vi "20TMonitor.vi"() -> ()   [LabVIEW 2019]
uses:
  Utility/Monitor Communication/Gustav/20T_Cluster.ctl
  Instrument_Setup.vi
  Global/Global Variables/Data_Display_global.vi
  Equipment/Mercury iXX/Public/Libraries/Magnet/Open/Open Magnet Device.vi
  Equipment/Mercury iXX/Public/Libraries/Magnet/Signals/Read/Persistant Field (Read).vi
  Equipment/Mercury iXX/Public/Libraries/Magnet/Signals/Read/Field (Read).vi
  Equipment/Mercury iXX/Public/Libraries/Magnet/Signals/Read/Voltage (Read).vi
  Equipment/Mercury iXX/Public/Libraries/Lambda/Open/Open Lambda Device.vi
  Equipment/Mercury iXX/Public/Libraries/Lambda/Signals/Read/Lambda Pressure (Read).vi
  Equipment/Mercury iXX/Public/Libraries/Lambda/Signals/Read/Lambda Valve Open Percent (Read).vi
  Equipment/Mercury iXX/Public/Libraries/Magnet/Signals/Read/Switch Heater Status (Read).vi
  Equipment/Mercury iXX/Public/Libraries/Magnet/Configuration/Read/PSU Action Status (Read).vi
  Equipment/Mercury iXX/Public/Libraries/Magnet/Configuration/Read/PSU Status (Read).vi
  Equipment/Mercury iXX/Public/Libraries/Magnet/Signals/Read/Target Field (Read).vi
  Equipment/Mercury iXX/Public/Libraries/Magnet/Signals/Read/Target Field Rate (Read).vi
  Equipment/Mercury iXX/Public/Libraries/Temperature/Open/Open Temperature Device.vi
  Equipment/Mercury iXX/Public/Libraries/Temperature/Signals/Read/Temperature (Read).vi
  Utility/Monitor Communication/sub-vis/20T_Open_Queue.vi
  Utility/Gustav/20T_Set_Rate.vi
  Utility/Gustav/20T_Go_To_Set.vi
  Utility/Gustav/20T_Go_To_Zero.vi
  Utility/Gustav/20T_Set_Hold.vi
  Utility/Gustav/20T_Set_Clamp.vi
  Equipment/Mercury iXX/Mercury iXX.lvlib
  Equipment/Mercury iXX/Public/Libraries/Magnet.lvlib
  Equipment/Mercury iXX/Public/Libraries/Lambda.lvlib
  Equipment/Mercury iXX/Public/Libraries/Temperature.lvlib
panel:
  out "20 T Magnet control":T1={"Clamp"=FALSE, "Switch Heater"=FALSE, "Go to Zero"=FALSE, "Go to set"=FALSE, "Go to Hold"=FALSE, "Clamped"=FALSE, "Hold"=FALSE, "Set"=FALSE, "Zero"=FALSE, "Magnet (T)"=0.0, "Leads (T)"=0.0, "Magnet T (K)"=3.4572, "Switch"=FALSE, "Target Field (T)"=3.4572, "Field Setpoint (T)"=3.4572, "Rate Setpoint (T/min)"=0.0, "Set Rate"=FALSE, "Rate\n(T/min) "=3.4572, "lambda NV (%)"=3.4572, "lambda p (mbar)"=3.4572, "lambda-Control"=FALSE, "Activate lambda control"=FALSE, "lambda NV  SP"=3.4572, "Set lambda NV"=FALSE, "PSU Status"="", "PSU\nVoltage"=3.4572} {"PSU\nVoltage" format="%.3f"; "lambda NV  SP" format="%.1f"; "lambda p (mbar)" format="%.1f"; "lambda NV (%)" scale=0.0..100.0; "Rate\n(T/min)" format="%.3f"; "Rate Setpoint (T/min)" format="%6.3f"; "Field Setpoint (T)" format="%6.3f"; "Target Field (T)" format="%.3f"; "Magnet T (K)" format="%4.3f"; "Leads (T)" format="%.3f"; "Magnet (T)" format="%.3g"}
  # "20 T"
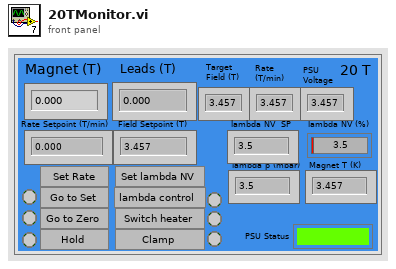
[diagram p1: front panel]
types:
  T1 = typedef "20T_Cluster.ctl" = cluster{"Clamp":bool, "Switch Heater":bool, "Go to Zero":bool, "Go to set":bool, "Go to Hold":bool, "Clamped":bool, "Hold":bool, "Set":bool, "Zero":bool, "Magnet (T)":dbl, "Leads (T)":dbl, "Magnet T (K)":dbl, "Switch":bool, "Target Field (T)":dbl, "Field Setpoint (T)":dbl, "Rate Setpoint (T/min)":dbl, "Set Rate":bool, "Rate\n(T/min) ":dbl, "lambda NV (%)":dbl, "lambda p (mbar)":dbl, "lambda-Control":bool, "Activate lambda control":bool, "lambda NV  SP":dbl, "Set lambda NV":bool, "PSU Status":string, "PSU\nVoltage":dbl}
  T2 = typedef "Mercury iXX.lvlib/Mercury Reference.ctl" = cluster{"Comms":refnum<visa-resource-name>, "Device ID":string[], "Comms Layer":T3, "Command":string, "Query reference":T4}
  T3 = typedef "Mercury iXX.lvlib/Comms Transport Layer.ctl" = enum16{"Ethernet TCP/IP", "USB", "ISOBus - RS-232", "GPIB"}
  T4 = typedef "Mercury iXX.lvlib/Query Dynamic Reference.ctl" = refnum<vi>
  T5 = typedef "Mercury iXX.lvlib/Magnet.lvlib/PSU Actions.ctl" = string
  T6 = typedef "20T_Control.ctl" = cluster{"Clamp":bool, "Switch Heater":bool, "Go to Zero":bool, "Go to Set":bool, "Go to Hold":bool, "Field Setpoint (T)":dbl, "Rate Setpoint (T/min)":dbl, "Set Rate":bool, "Activate lambda control":bool, "Set lambda NV":bool, "lambda NV  SP":dbl}
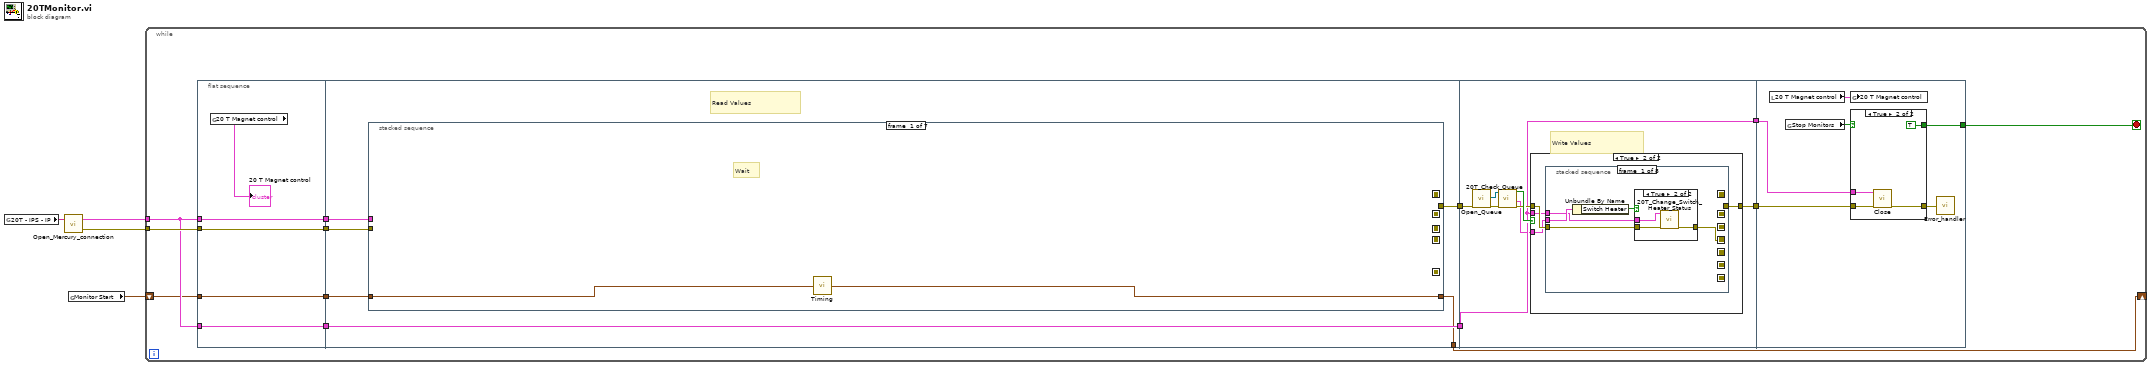
[diagram p0: block diagram]
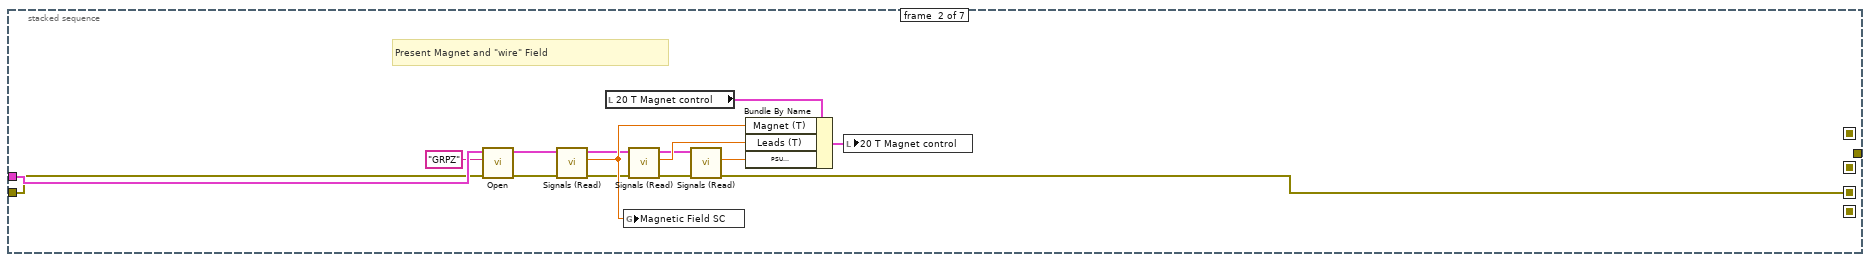
[diagram p2: hidden frame]
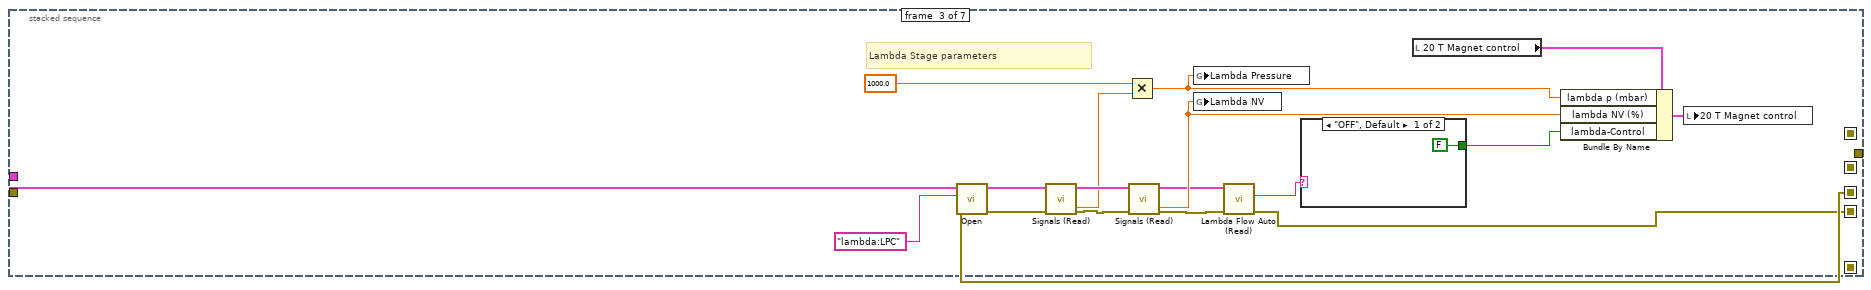
[diagram p3: hidden frame]
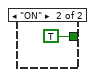
[diagram p4: hidden frame]
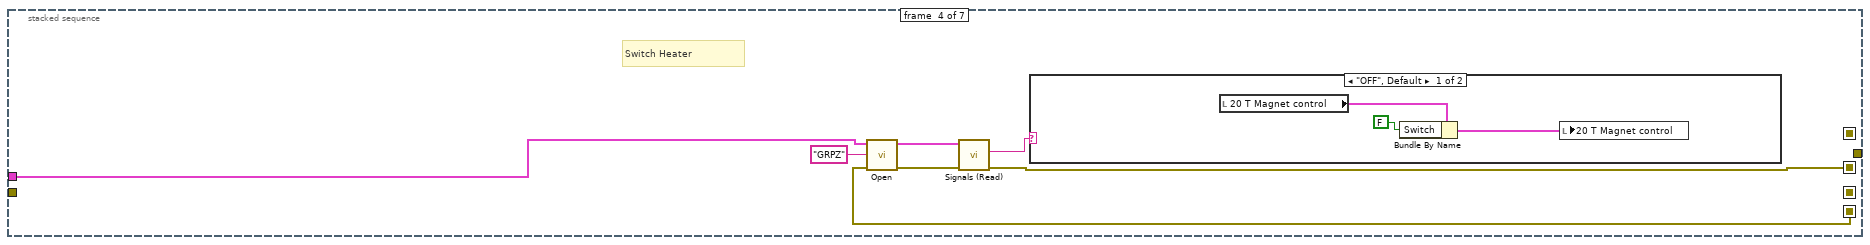
[diagram p5: hidden frame]
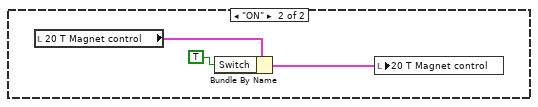
[diagram p6: hidden frame]
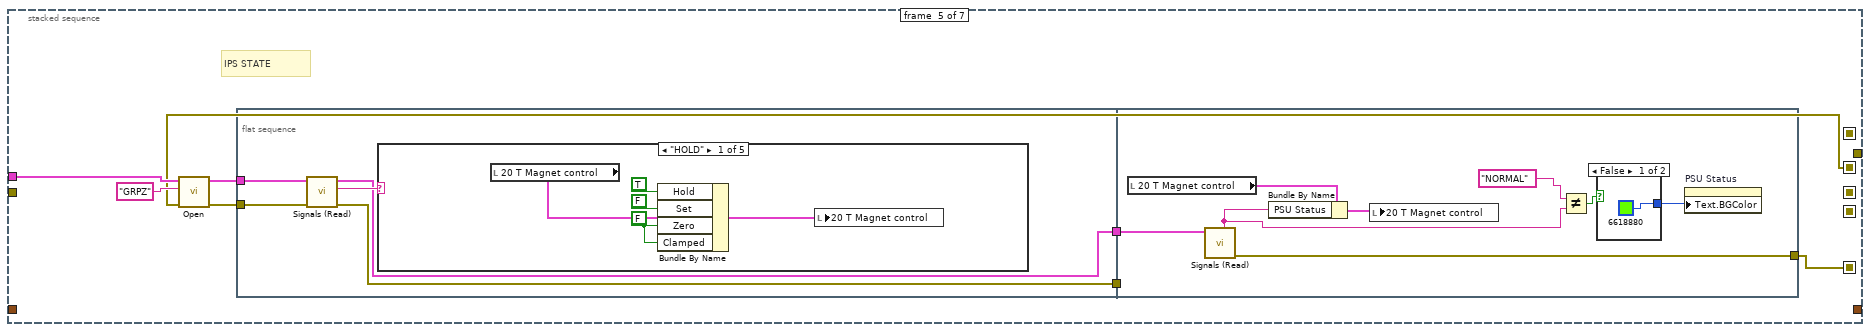
[diagram p7: hidden frame]
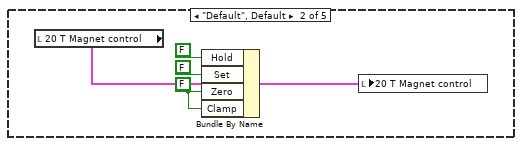
[diagram p8: hidden frame]
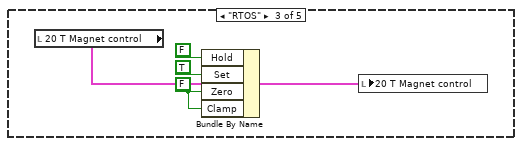
[diagram p9: hidden frame]
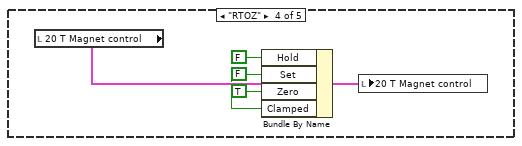
[diagram p10: hidden frame]
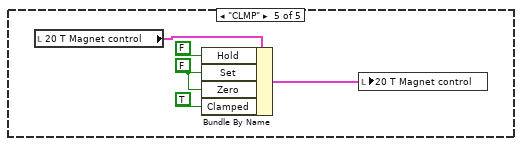
[diagram p11: hidden frame]
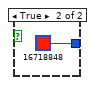
[diagram p12: hidden frame]
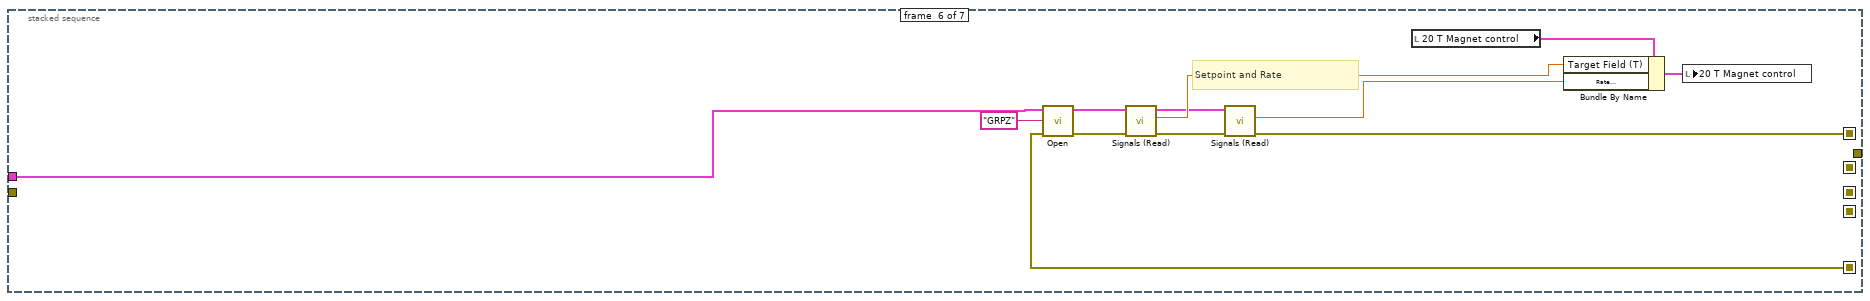
[diagram p13: hidden frame]
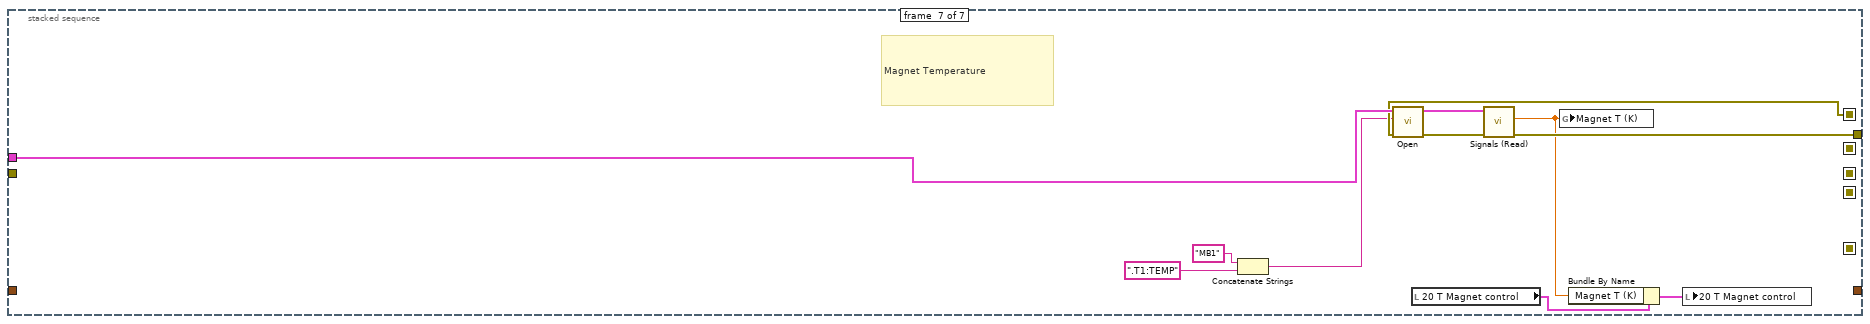
[diagram p14: hidden frame]
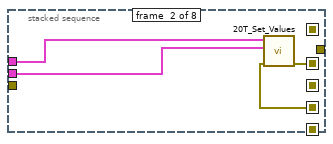
[diagram p17: hidden frame]
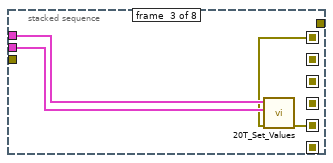
[diagram p18: hidden frame]
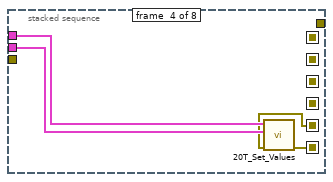
[diagram p19: hidden frame]
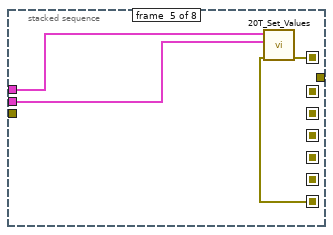
[diagram p20: hidden frame]
diagram:
  n1 = global read "Instrument_Setup.vi" "20T - IPS - IP"() -> (w4:string)
  n2 = call "Open_Mercury_connection.vi"("IP Address"=w4) -> ("error out"=w3:errorcluster, "Mercury Reference Out"=w2:T2)  [unwired: 1 in]
  n3 = global read "Data_Display_global.vi" "Monitor Start"() -> (w1:timestamp)
  n4 = while {
    tunnel: w3 -> [w15]
    tunnel: w2 -> [w14]
    shift-right: [w11] -> _
    shift-left: w1 -> [w12]
    stop <- w17 stop-if-true
    n5 = flat-sequence {
      tunnel: w12 -> [w19]
      tunnel: w14 -> [w20]
      tunnel: w14 -> [w21]
      tunnel: w15 -> [w22]
      tunnel: [w22] -> w10
      tunnel: [w21] -> w9
      tunnel: [w20] -> w8
      tunnel: [w19] -> w7
      tunnel: [w28] -> w16
      tunnel: [w25] -> w13
      tunnel: [w24] -> w11
      tunnel: w10 -> [w27]
      tunnel: w9 -> [w26]
      tunnel: w8 -> [w25]
      tunnel: w7 -> [w23]
      tunnel: [w151] -> w6
      tunnel: [w157] -> w5
      tunnel: w16 -> [w154]
      tunnel: w13 -> [w151]
      tunnel: w6 -> [w204]
      tunnel: w5 -> [w203]
      tunnel: [w201] -> w17
      frame #0 {
        n6 = global read "Data_Display_global.vi" "20 T Magnet control"() -> (→"20 T Magnet control":T1)
      }
      frame #1 {
        # "Read Values"
        n7 = stacked-sequence {
          seq-local: [_ w34 _ _ _ _ _] -> [_ _ w61 _ _ _ _]
          seq-local: [_ _ w47 _ _ _ _] -> [_ _ _ w68 _ _ _]
          seq-local: [_ _ _ w67 _ _ _] -> [_ _ _ _ w82 _ _]
          seq-local: [_ _ _ _ w79 _ _] -> [_ _ _ _ _ w134 _]
          seq-local: [_ _ _ _ _ w129 _] -> [_ _ _ _ _ _ w143]
          tunnel: w26 -> [_ w43 w51 w70 w84 w136 w147]
          tunnel: w27 -> [_ w42 _ _ _ _ _]
          tunnel: [_ _ _ _ _ _ w146] -> w28
          tunnel: [w30 _ _ _ _ _ _] -> w24
          tunnel: w23 -> [w29 _ _ _ _ _ _]
          frame #0 {
            # "Wait"
            n8 = call "Timing.vi"("start time (s)"=w29) -> ("last reading (s)"=w30:timestamp)
          }
          frame #1 {
            # "Present Magnet and \"wire\" Field"
            n9 = call-poly "Open.vi"("error in (no error)"=w42, "Device Identifier"="GRPZ", "Mercury Reference In"=w43) -> ("error out"=w45:errorcluster, "Mercury Reference Out"=w44:T2)  [unwired: 1 in, 6 out]
            n10 = call-poly "Signals (Read).vi"("error in"=w45, "Mercury Reference In"=w44) -> ("error out"=w35:errorcluster, "Persistant Field"=w38:dbl, "Mercury Reference Out"=w37:T2)  [unwired: 5 in, 2 out]
            n11 = local read "20 T Magnet control"() -> (w40:T1)
            n12 = global write "Data_Display_global.vi" "Magnetic Field SC"(w38) -> ()
            n13 = call-poly "Signals (Read).vi"("error in"=w35, "Mercury Reference In"=w37) -> ("error out"=w33:errorcluster, "Field"=w36:dbl, "Mercury Reference Out"=w32:T2)  [unwired: 5 in, 2 out]
            n14 = call-poly "Signals (Read).vi"("error in"=w33, "Mercury Reference In"=w32) -> ("error out"=w34:errorcluster, "Voltage"=w31:dbl)  [unwired: 5 in, 3 out]
            n15 = Bundle By Name(cluster=w40, "Magnet (T)"=w38, "Leads (T)"=w36, "PSU\nVoltage"=w31) -> (w39:T1)
            n16 = local write "20 T Magnet control"(w39) -> ()
          }
          frame #2 {
            # "Lambda Stage parameters"
            n17 = call-poly "Open.vi"("error in (no error)"=w61, "Device Identifier"="lambda:LPC", "Mercury Reference In"=w51) -> ("error out"=w63:errorcluster, "Mercury Reference Out"=w62:T2)  [unwired: 1 in, 6 out]
            n18 = call-poly "Signals (Read).vi"("error in"=w63, "Mercury Reference In"=w62) -> ("error out"=w58:errorcluster, "Pressure"=w55:dbl, "Mercury Reference Out"=w57:T2)  [unwired: 5 in, 2 out]
            n19 = Multiply(x=1000.0, y=w55) -> (x*y=w52:dbl)
            n20 = call-poly "Signals (Read).vi"("error in"=w58, "Mercury Reference In"=w57) -> ("error out"=w48:errorcluster, "Open"=w53:dbl, "Mercury Reference Out"=w49:T2)  [unwired: 5 in, 2 out]
            n21 = global write "Data_Display_global.vi" "Lambda Pressure"(w52) -> ()
            n22 = global write "Data_Display_global.vi" "Lambda NV"(w53) -> ()
            n23 = call "Lambda Flow Auto (Read).vi"("error in"=w48, "Mercury Reference In"=w49) -> ("error out"=w47:errorcluster, "Lambda Auto"=w46:string)  [unwired: 6 in, 2 out]
            n24 = case shown="\"OFF\", Default" w46 {
              tunnel: [FALSE TRUE] -> w50
              frame "OFF", Default {
              }
              frame "ON" {
              }
            }
            n25 = local read "20 T Magnet control"() -> (w60:T1)
            n26 = Bundle By Name(cluster=w60, "lambda p (mbar)"=w52, "lambda NV (%)"=w53, "lambda-Control"=w50) -> (w59:T1)
            n27 = local write "20 T Magnet control"(w59) -> ()
          }
          frame #3 {
            # "Switch Heater"
            n28 = call-poly "Open.vi"("error in (no error)"=w68, "Device Identifier"="GRPZ", "Mercury Reference In"=w70) -> ("error out"=w72:errorcluster, "Mercury Reference Out"=w71:T2)  [unwired: 1 in, 6 out]
            n29 = call-poly "Signals (Read).vi"("error in"=w72, "Mercury Reference In"=w71) -> ("error out"=w67:errorcluster, "Switch Heater Status"=w66:string)  [unwired: 6 in, 2 out]
            n30 = case shown="\"OFF\", Default" w66 {
              frame "OFF", Default {
                n31 = local read "20 T Magnet control"() -> (w73:T1)
                n32 = Bundle By Name(cluster=w73, "Switch"=FALSE) -> (w75:T1)
                n33 = local write "20 T Magnet control"(w75) -> ()
              }
              frame "ON" {
                n34 = local read "20 T Magnet control"() -> (w77:T1)
                n35 = Bundle By Name(cluster=w77, "Switch"=TRUE) -> (w78:T1)
                n36 = local write "20 T Magnet control"(w78) -> ()
              }
            }
          }
          frame #4 {
            # "IPS STATE"
            n37 = call-poly "Open.vi"("error in (no error)"=w82, "Device Identifier"="GRPZ", "Mercury Reference In"=w84) -> ("error out"=w86:errorcluster, "Mercury Reference Out"=w85:T2)  [unwired: 1 in, 6 out]
            n38 = flat-sequence {
              tunnel: w86 -> [w91]
              tunnel: w85 -> [w90]
              tunnel: [w88] -> w81
              tunnel: [w87] -> w80
              tunnel: w81 -> [w123]
              tunnel: w80 -> [_]
              tunnel: [w124] -> w79
              frame #0 {
                n39 = call-poly "Signals (Read).vi"("error in"=w91, "Mercury Reference In"=w90) -> ("error out"=w87:errorcluster, "PSU Act Stat"=w89:T5, "Mercury Reference Out"=w88:T2)  [unwired: 6 in, 1 out]
                n40 = case shown="\"HOLD\"" w89 {
                  frame "HOLD" {
                    w92 = FALSE
                    n41 = local read "20 T Magnet control"() -> (w96:T1)
                    n42 = Bundle By Name(cluster=w96, "Hold"=TRUE, "Set"=FALSE, "Zero"=w92, "Clamped"=w92) -> (w95:T1)
                    n43 = local write "20 T Magnet control"(w95) -> ()
                  }
                  frame "Default", Default {
                    w97 = FALSE
                    n44 = local read "20 T Magnet control"() -> (w101:T1)
                    n45 = Bundle By Name(cluster=w101, "Hold"=FALSE, "Set"=FALSE, "Zero"=w97, "Clamp"=w97) -> (w100:T1)
                    n46 = local write "20 T Magnet control"(w100) -> ()
                  }
                  frame "RTOS" {
                    w102 = FALSE
                    n47 = local read "20 T Magnet control"() -> (w106:T1)
                    n48 = Bundle By Name(cluster=w106, "Hold"=FALSE, "Set"=TRUE, "Zero"=w102, "Clamp"=w102) -> (w105:T1)
                    n49 = local write "20 T Magnet control"(w105) -> ()
                  }
                  frame "RTOZ" {
                    w107 = FALSE
                    n50 = local read "20 T Magnet control"() -> (w111:T1)
                    n51 = Bundle By Name(cluster=w111, "Hold"=FALSE, "Set"=w107, "Zero"=TRUE, "Clamped"=w107) -> (w110:T1)
                    n52 = local write "20 T Magnet control"(w110) -> ()
                  }
                  frame "CLMP" {
                    w112 = FALSE
                    n53 = local read "20 T Magnet control"() -> (w116:T1)
                    n54 = Bundle By Name(cluster=w116, "Hold"=FALSE, "Set"=w112, "Zero"=w112, "Clamped"=TRUE) -> (w115:T1)
                    n55 = local write "20 T Magnet control"(w115) -> ()
                  }
                }
              }
              frame #1 {
                n56 = local read "20 T Magnet control"() -> (w122:T1)
                n57 = call-poly "Signals (Read).vi"("Mercury Reference In"=w123) -> ("error out"=w124:errorcluster, "Status"=w120:string)  [unwired: 5 in, 4 out]
                n58 = Bundle By Name(cluster=w122, "PSU Status"=w120) -> (w121:T1)
                n59 = local write "20 T Magnet control"(w121) -> ()
                n60 = Not Equal?(x="NORMAL", y=w120) -> (x != y?=w118:bool)
                n61 = case shown="False" w118 {
                  tunnel: [u32 6618880 u32 16718848] -> w117
                  frame False {
                  }
                  frame True {
                  }
                }
                n62 = property on="PSU Status" class="Str"("Text.BGColor"=w117) -> ()  [unwired: 2 in, 2 out]
              }
            }
          }
          frame #5 {
            # "Setpoint and Rate"
            n63 = call-poly "Open.vi"("error in (no error)"=w134, "Device Identifier"="GRPZ", "Mercury Reference In"=w136) -> ("error out"=w138:errorcluster, "Mercury Reference Out"=w137:T2)  [unwired: 1 in, 6 out]
            n64 = call-poly "Signals (Read).vi"("error in"=w138, "Mercury Reference In"=w137) -> ("error out"=w130:errorcluster, "Target Field"=w131:dbl, "Mercury Reference Out"=w128:T2)  [unwired: 5 in, 2 out]
            n65 = call-poly "Signals (Read).vi"("error in"=w130, "Mercury Reference In"=w128) -> ("error out"=w129:errorcluster, "Target Field Rate"=w127:dbl)  [unwired: 5 in, 3 out]
            n66 = local read "20 T Magnet control"() -> (w133:T1)
            n67 = Bundle By Name(cluster=w133, "Target Field (T)"=w131, "Rate\n(T/min)"=w127) -> (w132:T1)
            n68 = local write "20 T Magnet control"(w132) -> ()
          }
          frame #6 {
            # "Magnet Temperature"
            n69 = Concatenate Strings("MB1", ".T1:TEMP" ("Device Identifier")) -> (w140:string)
            n70 = call-poly "Open.vi"("error in (no error)"=w143, "Device Identifier"=w140, "Mercury Reference In"=w147) -> ("error out"=w149:errorcluster, "Mercury Reference Out"=w148:T2)  [unwired: 1 in, 6 out]
            n71 = local read "20 T Magnet control"() -> (w145:T1)
            n72 = call-poly "Signals (Read).vi"("error in"=w149, "Mercury Reference In"=w148) -> ("error out"=w146:errorcluster, "Temperature"=w139:dbl)  [unwired: 5 in, 3 out]
            n73 = global write "Data_Display_global.vi" "Magnet T (K)"(w139) -> ()
            n74 = Bundle By Name(cluster=w145, "Magnet T (K)"=w139) -> (w144:T1)
            n75 = local write "20 T Magnet control"(w144) -> ()
          }
        }
      }
      frame #2 {
        # "Write Values"
        n76 = call-poly "Open_Queue.vi"("error in (no error)"=w154) -> ("error out"=w153:errorcluster, "queue out"=w156:refnum<queue>)  [unwired: 9 in]
        n77 = call "20T_Check_Queue.vi"("error in (no error)"=w153, "queue"=w156) -> ("error out"=w152:errorcluster, "Control"=w150:T6, "New Entries?"=w155:bool)  [unwired: 6 in]
        n78 = case shown="True" w155 {
          tunnel: w152 -> [w158 w162]
          tunnel: [w158 w159] -> w157
          tunnel: w151 -> [_ w161]
          tunnel: w150 -> [_ w160]
          frame False {
          }
          frame True {
            n79 = stacked-sequence {
              seq-local: [_ w173 _ _ _ _ _ _] -> [_ _ w177 _ _ _ _ _]
              seq-local: [_ _ w176 _ _ _ _ _] -> [_ _ _ w181 _ _ _ _]
              seq-local: [_ _ _ w180 _ _ _ _] -> [_ _ _ _ w185 _ _ _]
              seq-local: [_ _ _ _ w184 _ _ _] -> [_ _ _ _ _ w189 _ _]
              seq-local: [w163 _ _ _ _ _ _ _] -> [_ w172 _ _ _ _ _ _]
              seq-local: [_ _ _ _ _ w188 _ _] -> [_ _ _ _ _ _ w195 _]
              seq-local: [_ _ _ _ _ _ w192 _] -> [_ _ _ _ _ _ _ w199]
              tunnel: w162 -> [w165 _ _ _ _ _ _ _]
              tunnel: [_ _ _ _ _ _ _ w198] -> w159
              tunnel: w161 -> [w164 w175 w179 w183 w187 w191 w193 w196]
              tunnel: w160 -> [w167 w174 w178 w182 w186 w190 w194 w197]
              frame #0 {
                n80 = Unbundle By Name(w167) -> ("Switch Heater"=w166:bool)
                n81 = case shown="True" w166 {
                  tunnel: w165 -> [w168 w170]
                  tunnel: [w168 w169] -> w163
                  tunnel: w164 -> [_ w171]
                  frame False {
                  }
                  frame True {
                    n82 = call "20T_Change_Switch_Heater_Status.vi"("error in (no error)"=w170, "Mercury Reference In"=w171) -> ("error out"=w169:errorcluster)  [unwired: 9 in]
                  }
                }
              }
              frame #1 {
                n83 = call-poly "20T_Set_Values.vi"("error in (no error)"=w172, "20T Control"=w174, "Mercury Reference In"=w175) -> ("error out"=w173:errorcluster)  [unwired: 8 in]
              }
              frame #2 {
                n84 = call-poly "20T_Set_Values.vi"("error in (no error)"=w177, "20T Control"=w178, "Mercury Reference In"=w179) -> ("error out"=w176:errorcluster)  [unwired: 8 in]
              }
              frame #3 {
                n85 = call-poly "20T_Set_Values.vi"("error in (no error)"=w181, "20T Control"=w182, "Mercury Reference In"=w183) -> ("error out"=w180:errorcluster)  [unwired: 8 in]
              }
              frame #4 {
                n86 = call-poly "20T_Set_Values.vi"("error in (no error)"=w185, "20T Control"=w186, "Mercury Reference In"=w187) -> ("error out"=w184:errorcluster)  [unwired: 8 in]
              }
              frame #5 {
                n87 = call-poly "20T_Set_Values.vi"("error in (no error)"=w189, "20T Control"=w190, "Mercury Reference In"=w191) -> ("error out"=w188:errorcluster)  [unwired: 8 in]
              }
              frame #6 {
                n88 = call "20T_Change_lambda_Control_Status.vi"("error in (no error)"=w195, "20 T Magnet control"=w194, "Mercury Reference In"=w193) -> ("error out"=w192:errorcluster)  [unwired: 8 in]
              }
              frame #7 {
                n89 = call "20T_Set_lambda_NV.vi"("error in (no error)"=w199, "20T Control"=w197, "Mercury Reference In"=w196) -> ("error out"=w198:errorcluster)  [unwired: 8 in]
              }
            }
          }
        }
      }
      frame #3 {
        n90 = local read "20 T Magnet control"() -> (w200:T1)
        n91 = global read "Data_Display_global.vi" "Stop Monitors"() -> (w205:bool)
        n92 = global write "Data_Display_global.vi" "20 T Magnet control"(w200) -> ()
        n93 = case shown="True" w205 {
          tunnel: w204 -> [_ w211]
          tunnel: w203 -> [w207 w210]
          tunnel: [w207 w209] -> w202
          tunnel: [FALSE TRUE] -> w201
          frame False {
          }
          frame True {
            n94 = call "Close.vi"("error in (no error)"=w210, "Mercury Reference"=w211) -> ("error out"=w209:errorcluster)  [unwired: 9 in]
          }
        }
        n95 = call "Error_handler.vi"("error constant"=w202) -> ()
      }
    }
  }
